vi "terminate.vi"(8 "error in (no error)":errorcluster, 11 "DL090430TriggeredExperimentController in":refnum<class "ExperimentControllerDL090430DAQmxTriggered.lvclass">) -> (0 "error out":errorcluster, 3 "DL090430TriggeredExperimentController out":refnum<class "ExperimentControllerDL090430DAQmxTriggered.lvclass">)   [LabVIEW 2010, in "ExperimentControllerDL090430DAQmxTriggered.lvclass"]
doc: "The dynamic dispatch version of this VI terminates the plug-in object by releasing all of its resources."
uses:
  ExperimentControllerDL090430DAQmxTriggered.lvclass
  ExperimentControllerDL090430DAQmxTriggered.lvclass/ExperimentControllerDL090430DAQmxTriggered.ctl
  GenericExperimentController/GenericExperimentController/GenericExperimentController.lvclass
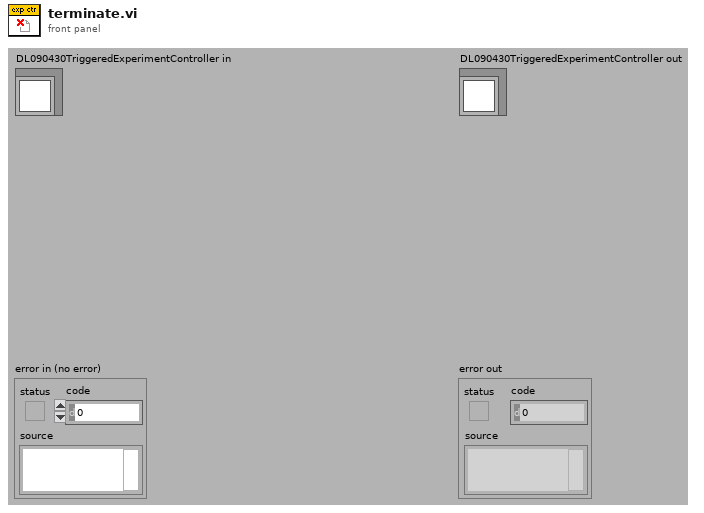
[diagram p1: front panel]
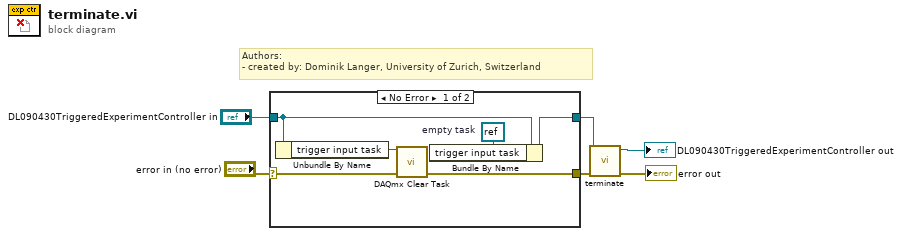
[diagram p0: block diagram]
diagram:
  # "Authors: \n- created by: Dominik Langer, University of Zurich, Switzerland"
  n1 = case shown="No Error" "error in (no error)" {
    selector: "error in (no error)" -> [w11 w13]
    tunnel: [w10 w13] -> w3
    tunnel: "DL090430TriggeredExperimentController in" -> [w9 w14]
    tunnel: [w8 w14] -> w1
    frame No Error {
      w7 = refnum<k21> refnum  # empty task
      n2 = Unbundle By Name(w9) -> ("trigger input task"=w12:refnum<k21>)
      n3 = call <vilib>:"DAQmx Clear Task.vi"("task in"=w12, "error in"=w11) -> ("error out"=w10:errorcluster)  [unwired: 13 out]
      n4 = Bundle By Name(cluster=w9, "trigger input task"=w7) -> (w8:refnum<class "ExperimentControllerDL090430DAQmxTriggered.lvclass">)
    }
    frame Error {
    }
  }
  n5 = call-parent "terminate.vi"("error in (no error)"=w3, "GenericPlugin in"=w1) -> ("error out"=→"error out":errorcluster, "GenericPlugin out"=→"DL090430TriggeredExperimentController out":refnum<class "ExperimentControllerDL090430DAQmxTriggered.lvclass">)  [unwired: 8 out]
